vi "Kalman Filter Laptop Demo.vi"() -> ()   [LabVIEW 2020]
uses:
  ctl/XY (Position-Velocity) Sensor Instance.ctl
  <vilib>/Analysis/Matrix/Datatypes/RealMatrix.ctl
  ctl/Dynamical System Templates.ctl
  <vilib>/Analysis/baseanly.llb/Real A x B.vi
  <vilib>/Analysis/Matrix/Numeric/Conversions/Matrix To Array - RM.vi
  <vilib>/Analysis/Matrix/Numeric/Add/Add - RM,RM.vi
  <vilib>/Analysis/Matrix/NI_Matrix.lvlib
  <vilib>/Analysis/NI_AALBase.lvlib
panel:
  out "Arcade Inputs":picture
  out "Predicted State":T1
  out "Estimated State":T1
  in  "Friction Standard Deviation":dbl=1.0000000000000002 format="%0.2f"
  in  "Friction":dbl=0.1
  out "Current State":T1
  out "Simulation":cluster{dbl[], dbl[]}[](graph)
  in  "State Estimate Standard Deviation":dbl=1.0
  in  "Sensors":T2[](array[typedef])
  in  "dt (s)":dbl=0.1
  # "Kalman Filter Demo:"
  # "How to Use:\n\n1.) Add the Sensors along with their\nrespective measurement uncertainties\n\n2.) Configure Friction Settings along with\nthe state estimate uncertainty\n\n3.) Run the simulation and move the\nrobot around using the joystick"
  # "This demo models the pose tracking of a rigid body moving in 2 dimensions. Using noisy position and velocity sensors, this demo illustrates how to fuse these sensor measurements to estimate the rigid body's pose"
  # "Front (1)"
  # "Left (-1)"
  # "Right (1)"
  # "Back (-1)"
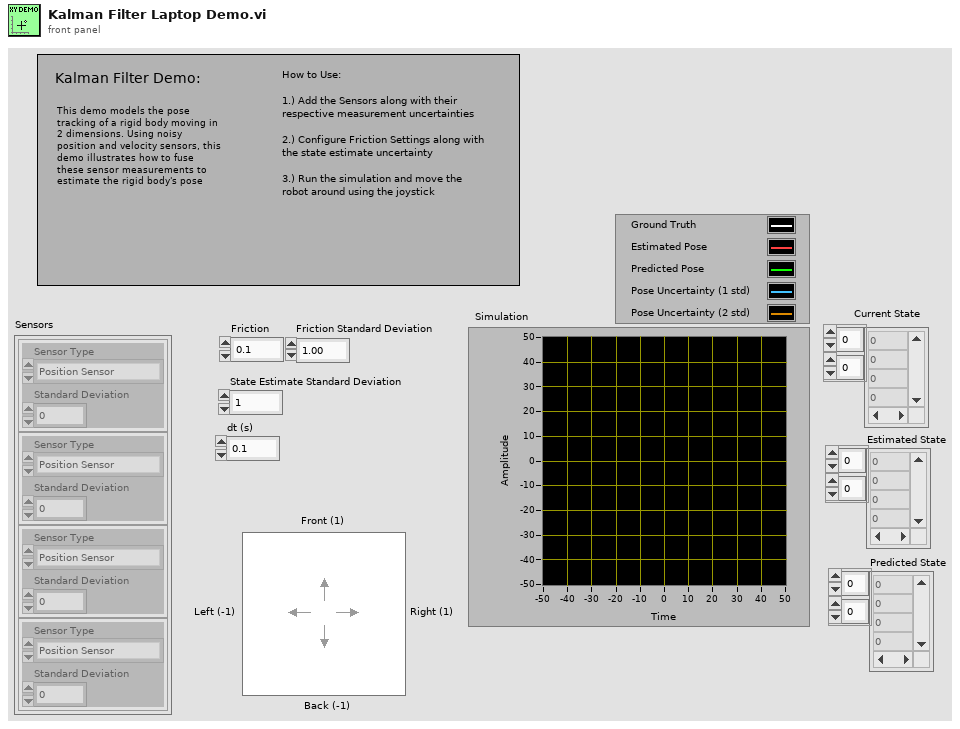
[diagram p1: front panel]
types:
  T1 = typedef "NI_Matrix.lvlib/RealMatrix.ctl" = dbl[][]
  T2 = typedef "XY (Position-Velocity) Sensor Instance.ctl" = cluster{"Sensor Type":enum16{"Position Sensor", "Velocity Sensor"}, "Standard Deviation":dbl}
  T3 = typedef "Dynamical System Matrices.ctl" = cluster{"F (State Transition Matrix)":T1, "G (Control Matrix)":T1, "H (Observation Matrix)":T1, "Q (Process Noise Uncertainty)":T1, "R (Measurement Uncertainty)":T1}
  T4 = typedef "Kalman Filter Instance.ctl" = cluster{"Current State":T1, "Current Covariance":T1, "Predicted State":T1, "Predicted Covariance":T1, "Dynamical System Matrices":T3}
  T5 = typedef "LVBoundsTypeDef.ctl" = cluster{"Width":u32, "Height":u32}
  T6 = typedef "Dynamical System Templates.ctl" = enum16{"XY Point Mass"}
  T7 = typedef "LVMouseTypeDef.ctl" = cluster{"Mouse Position":cluster{"X":i32, "Y":i32}, "Mouse Modifiers":cluster{"Button Down":bool, "Shift Mod":bool, "Menu Mod":bool, "Option Mod":bool}}
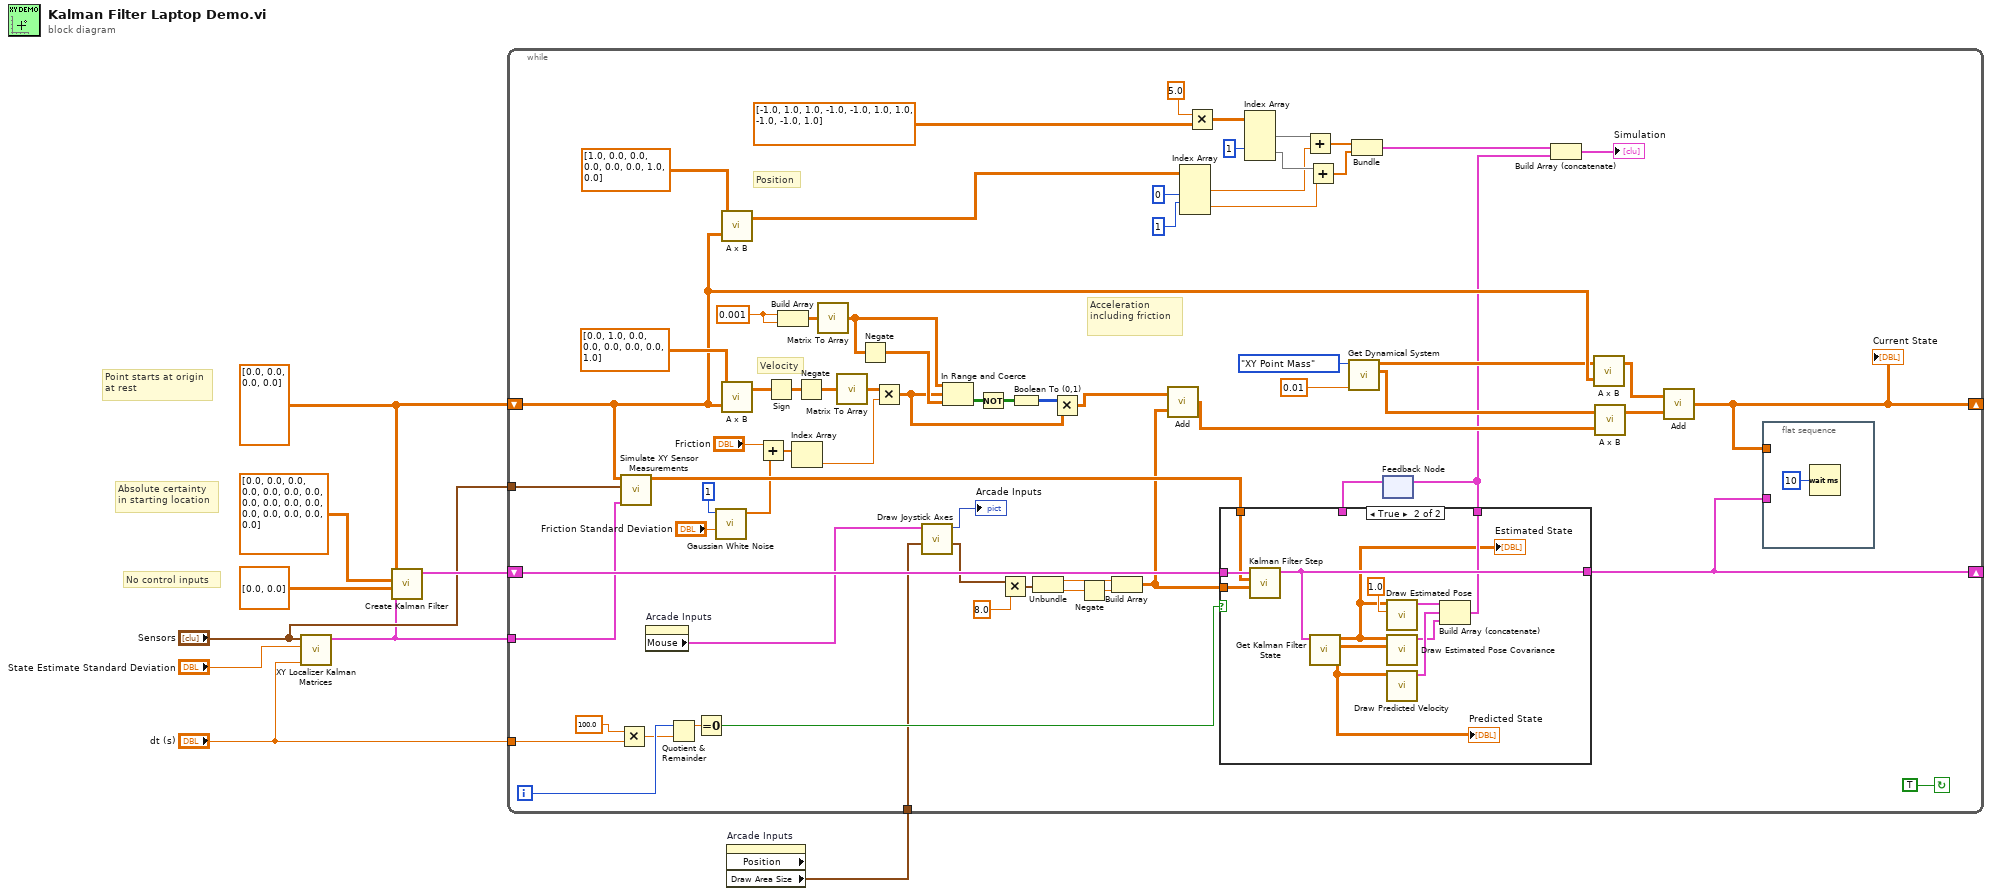
[diagram p0: block diagram]
diagram:
  w5 = T1 [[0.0], [0.0], [0.0], [0.0]] ("Guessed Initial State")
  # "No control inputs"
  # "Absolute certainty\nin starting location"
  # "Point starts at origin\nat rest"
  n1 = call "XY Localizer Kalman Matrices.vi"("dt (s)"="dt (s)", "State Estimate Standard Deviation"="State Estimate Standard Deviation", "Sensors"="Sensors") -> ("Dynamical System Matrices"=w3:T3)  [unwired: 8 in]
  n2 = call "Create Kalman Filter.vi"("Dynamical System Matrices"=w3, "Initial Control Input"=T1 [[0.0], [0.0]], "Guessed Initial Covariance"=T1 [[0.0, 0.0, 0.0, 0.0], [0.0, 0.0, 0.0, 0.0], [0.0, 0.0, 0.0, 0.0], [0.0, 0.0, 0.0, 0.0]], "Guessed Initial State"=w5) -> ("Kalman Filter"=w6:T4)  [unwired: 7 in]
  n3 = property on="Arcade Inputs" class="Pict" props=["Position", "Draw Area Size"]() -> ("Draw Area Size"=w1:T5)  [unwired: 2 in, 3 out]
  n4 = while {
    shift-right: [w28] -> _
    shift-left: w6 -> [w78]
    shift-right: [w29] -> _
    shift-left: w5 -> [w54]
    tunnel: "Sensors" -> [w77]
    tunnel: w3 -> [w55]
    tunnel: "dt (s)" -> [w70]
    tunnel: w1 -> [w19]
    i -> [w27]
    stop <- TRUE continue-if-true
    w35 = 0.001 ("Real Matrix Element")
    w34 = 0 ("disabled index (col)")
    # "Acceleration including friction"
    # "Velocity"
    # "Position"
    n5 = Multiply(x=100.0, y=w70) -> (x*y=w26:dbl)
    n6 = call "Simulate XY Sensor Measurements.vi"("Dynamical System Matrices"=w55, "Sensors"=w77, "Current State"=w54) -> ("Observations"=w75:T1)  [unwired: 8 in]
    n7 = property on="Arcade Inputs" class="Pict"() -> ("Mouse"=w11:T7)  [unwired: 2 in, 2 out]
    n8 = Quotient & Remainder(x=w27, y=w26) -> (x-y*floor(x/y)=w25:dbl)  [unwired: 1 out]
    n9 = Equal To 0?(x=w25) -> (x = 0?=w23:bool)
    n10 = call <vilib>:"Gaussian White Noise.vi"("standard deviation"="Friction Standard Deviation", "samples"=1) -> ("Gaussian noise pattern"=w38:dbl[])  [unwired: 8 in, 1 out]
    n11 = call-poly <vilib>:"A x B.vi"("B"=w54, "A"=T1 [[1.0, 0.0, 0.0, 0.0], [0.0, 0.0, 1.0, 0.0]] ("Initial Control Input")) -> ("A x B"=w69:T1)  [unwired: 1 out]
    n12 = call-poly <vilib>:"A x B.vi"("B"=w54, "A"=T1 [[0.0, 1.0, 0.0, 0.0], [0.0, 0.0, 0.0, 1.0]] ("Initial Control Input")) -> ("A x B"=w71:T1)  [unwired: 1 out]
    n13 = Add(x="Friction", y=w38) -> (x+y=w37:dbl[])
    n14 = Sign(1:w71) -> (0:w72:T1)
    n15 = Build Array(w35, w35) -> (w49:T1)
    n16 = Index Array(array=w37) -> (element=w36:dbl)  [unwired: 1 in]
    n17 = Negate(x=w72) -> (-x=w57:T1)
    n18 = call-poly <vilib>:"Matrix To Array.vi"("Real Matrix"=w49) -> ("Real 2D Array"=w48:dbl[][])
    n19 = call-poly <vilib>:"Matrix To Array.vi"("Real Matrix"=w57) -> ("Real 2D Array"=w56:dbl[][])
    n20 = Negate(x=w48) -> (-x=w47:dbl[][])
    n21 = Multiply ("Multiply.vi")(x=w56, y=w36) -> (x*y=w43:dbl[][])
    n22 = call "Draw Joystick Axes.vi"("Size"=w19, "Mouse"=w11) -> ("JS Coords"=w15:cluster{"X":dbl, "Y":dbl}, "Arcade Inputs"=→"Arcade Inputs":picture)  [unwired: 8 in]
    n23 = In Range and Coerce(upper limit=w48, x=w43, lower limit=w47) -> (In Range?=w46:bool[][])  [unwired: 1 out]
    n24 = Not(x=w46) -> (.not. x?=w45:bool[][])
    n25 = Multiply(x=w15, y=8.0) -> (x*y=w16:cluster{"X":dbl, "Y":dbl})
    n26 = Boolean To (0,1)(Boolean=w45) -> (0, 1=w44:i16[][])
    n27 = Unbundle(w16) -> ("X"=w17:dbl, "Y"=w13:dbl)
    n28 = Multiply(x=w44, y=w43) -> (x*y=w42:dbl[][])
    n29 = Negate(x=w13) -> (-x=w12:dbl)
    n30 = Build Array(w17, w12) -> (w18:T1)
    n31 = call-poly <vilib>:"Add.vi"("Real Matrix B"=w18, "Real Matrix A"=w42) -> ("A + B"=w53:T1)
    n32 = Index Array(array=w69, index (row) #1=w34, index (col) #1=w34, index (row) #2=1 ("index (col)"), index (col) #2=w34) -> (element #1=w60:dbl, element #2=w61:dbl)
    n33 = Multiply(x=5.0, y=dbl[][] [[-1.0, 1.0, 1.0, -1.0, -1.0], [1.0, 1.0, -1.0, -1.0, 1.0]]) -> (x*y=w65:dbl[][])
    n34 = Index Array(array=w65, index (row) #2=1 ("index (row)")) -> (element #1=w63:dbl[], element #2=w62:dbl[])  [unwired: 3 in]
    n35 = Add(x=w63, y=w60) -> (x+y=w59:dbl[])
    n36 = Add(x=w62, y=w61) -> (x+y=w58:dbl[])
    n37 = call "Get Dynamical System.vi"("dt"=0.01, "Dynamical System"=Dynamical_System_Templates."XY Point Mass") -> ("G (Control Input Matrix)"=w21:T1, "F (State Transition Matrix)"=w22:T1)  [unwired: 8 in]
    n38 = Bundle(w59, w58) -> (w33:cluster{dbl[], dbl[]})  [unwired: 1 in]
    n39 = feedback #1() -> (w24:cluster{dbl[], dbl[]}[])  [unwired: 1 in]
    n40 = case shown="True" w23 {
      tunnel: w78 -> [w80 w92]
      tunnel: w75 -> [_ w91]
      tunnel: w18 -> [_ w90]
      tunnel: [w80 w88] -> w28
      tunnel: w24 -> [w79 _]
      tunnel: [w79 w83] -> w10
      frame False {
      }
      frame True {
        n41 = call "Kalman Filter Step.vi"("Control Input"=w90, "Observations"=w91, "Kalman Filter In"=w92) -> ("Kalman Filter Out"=w88:T4)  [unwired: 8 in]
        n42 = call "Get Kalman Filter State.vi"("Kalman Filter In"=w88) -> ("Predicted State"=w87:T1, "Current Covariance"=w82:T1, "Current State"=w81:T1)  [unwired: 7 in, 1 out]
        "Predicted State" <- w87
        "Estimated State" <- w81
        n43 = call "Draw Estimated Pose.vi"("Radius"=1.0, "State"=w81) -> ("Estimated Pose"=w86:cluster{dbl[], dbl[]})  [unwired: 9 in]
        n44 = call "Draw Estimated Pose Covariance.vi"("State Uncertainty"=w82, "Estimated State"=w81) -> ("Covariance Ellipses"=w84:cluster{dbl[], dbl[]}[])  [unwired: 9 in]
        n45 = call "Draw Predicted Velocity.vi"("State"=w87) -> ("Predicted Velocity"=w85:cluster{dbl[], dbl[]})  [unwired: 10 in]
        n46 = Build Array (concatenate)(w86, w85, w84) -> (w83:cluster{dbl[], dbl[]}[])
      }
    }
    n47 = feedback-in #1(w10) -> ()
    n48 = Build Array (concatenate)(w33, w10) -> (→"Simulation":cluster{dbl[], dbl[]}[])
    n49 = call-poly <vilib>:"A x B.vi"("B"=w54, "A"=w22) -> ("A x B"=w52:T1)  [unwired: 1 out]
    n50 = call-poly <vilib>:"A x B.vi"("B"=w53, "A"=w21) -> ("A x B"=w51:T1)  [unwired: 1 out]
    n51 = call-poly <vilib>:"Add.vi"("Real Matrix B"=w51, "Real Matrix A"=w52) -> ("A + B"=w29:T1)
    "Current State" <- w29
    n52 = flat-sequence {
      tunnel: w29 -> [_]
      tunnel: w28 -> [_]
      frame #0 {
        n53 = Wait (ms)(milliseconds to wait=u32 10) -> ()  [unwired: 1 out]
      }
    }
  }
